vi "LSCI332 SetManOutput.vi"(0 "VISA Rsrc":refnum<visa-resource-name>="GPIB0::12::INSTR", 5 "Boucle(1)":u32(ring) caption="Boucle" items=["Boucle 1", "Boucle 2"], 7 "ManOutput":dbl caption="Manual Output %" format="%#.2g", 11 "error in":errorcluster) -> (15 "error out":errorcluster)   [LabVIEW 2012]
doc: "Ce Vi envoie à l'instrument la valeur de \"Manual output\" de chauffage désiré, en %."
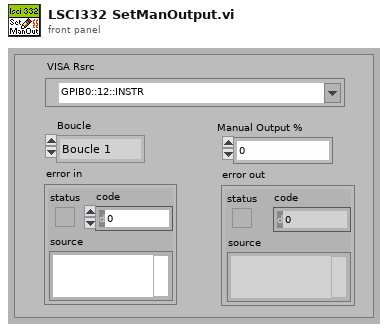
[diagram p1: front panel]
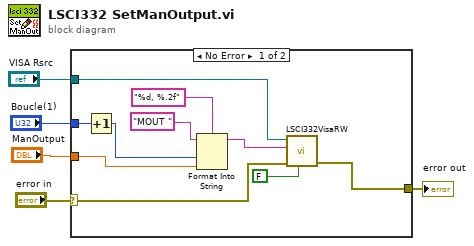
[diagram p0: block diagram]
diagram:
  n1 = case shown="No Error" "error in" {
    selector: "error in" -> [w14 w16]
    tunnel: [w11 w16] -> w5
    tunnel: "VISA Rsrc" -> [w15 _]
    tunnel: "ManOutput" -> [w9 _]
    tunnel: "Boucle(1)" -> [w10 _]
    frame No Error {
      n2 = Increment(x=w10) -> (x+1=w6:u32)
      n3 = Format Into String(format string="%d, %.2f", initial string="MOUT ", w6, w9) -> (resulting string=w7:string)  [unwired: 1 in, 1 out]
      n4 = call <userlib>:"LSCI332VisaRW.vi"("Lecture?(T)"=FALSE, "error in (no error)"=w14, "ChaineCom"=w7, "VISA Rsrc"=w15) -> ("error out"=w11:errorcluster)  [unwired: 3 in, 3 out]
    }
    frame Error {
    }
  }
  "error out" <- w5
